vi "Legend.vi"(8 "error in (no error)":errorcluster, 10 "Position":T1, 11 "Plot ID":T2 format="%x") -> (0 "error out":errorcluster, 3 "Plot ID Out":T2 format="%x")   [LabVIEW 2013, in "Advanced Plotting Toolkit.lvlib"]
doc: "Generate a legend describing the line, scatter, and bar objects plotted. Names to be displayed on the legend should be provided via the \"Legend Title\" terminal on the plotting VIs."
uses:
  Advanced Plotting Toolkit.lvlib
  typedefs/PlotID.ctl
  LegendPositions.ctl
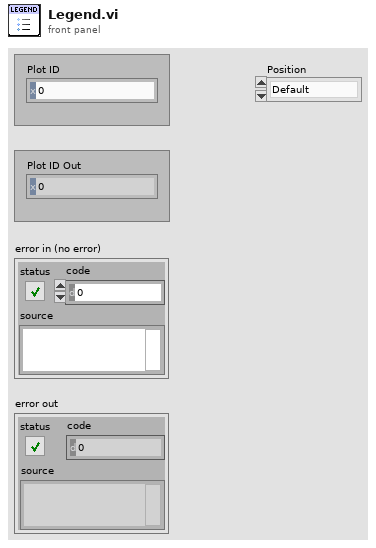
[diagram p1: front panel]
types:
  T1 = typedef "Advanced Plotting Toolkit.lvlib/LegendPositions.ctl" = enum16{"Default", "Top Right", "Top", "Top Left", "Left", "Bottom Left", "Bottom", "Bottom Right", "Right", "Center"}
  T2 = typedef "Advanced Plotting Toolkit.lvlib/PlotID.ctl" = i32
  T3 = typedef "Advanced Plotting Toolkit.lvlib/KeyValue.ctl" = cluster{"Key":string, "Value":string}
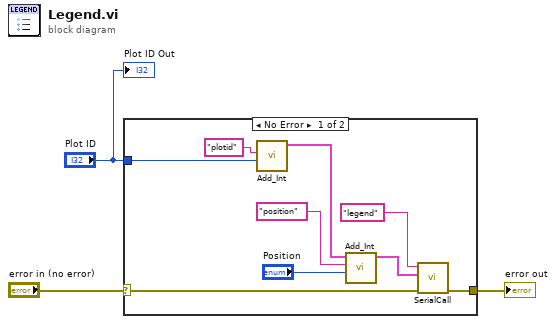
[diagram p0: block diagram]
diagram:
  n1 = case shown="No Error" "error in (no error)" {
    selector: "error in (no error)" -> [w10 w13]
    tunnel: "Plot ID" -> [w12 _]
    tunnel: [w9 w13] -> w1
    frame No Error {
      n2 = call "Add_Int.vi"("Value"=w12, "Key"="plotid") -> ("Keyword Array Out"=w4:T3[])  [unwired: 9 in]
      n3 = call "Add_Int.vi"("Value"="Position", "Key"="position", "Keyword Array"=w4) -> ("Keyword Array Out"=w6:T3[])  [unwired: 8 in]
      n4 = call "SerialCall.vi"("error in (no error)"=w10, "data"=w6, "Resource"="legend") -> ("error out"=w9:errorcluster)  [unwired: 7 in, 1 out]
    }
    frame Error {
    }
  }
  "error out" <- w1
  "Plot ID Out" <- "Plot ID"
